vi "_goop4.llb_Interface_ViServerCall.vi"(8 "error in (no error)":errorcluster, 10 "Caller VI ref (This is the interface VI's reference)":refnum<vi>, 11 "Interface In":refnum<class>) -> (0 "error out":errorcluster, 3 "Interface Out":refnum<class>)   [LabVIEW 2014]
doc: "This VI handles the call to the overriding VI in the class that implements this interface.\nUse the \"This VI\" reference and wirre that to the Caller VI ref control."
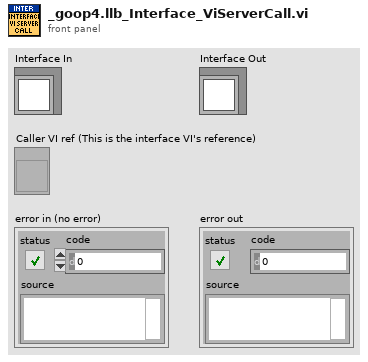
[diagram p1: front panel]
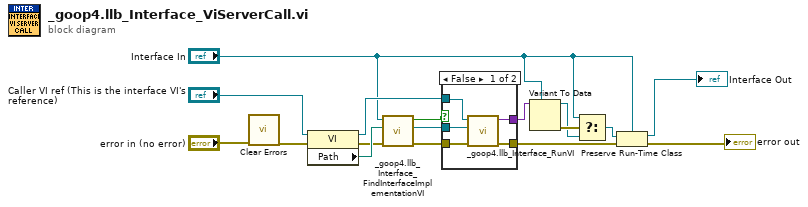
[diagram p0: block diagram]
diagram:
  n1 = call <vilib>:"Clear Errors.vi"("error in (no error)"="error in (no error)") -> ("error out"=w2:errorcluster)  [unwired: 5 in, 1 out]
  n2 = property class="VI"(reference="Caller VI ref (This is the interface VI's reference)", error in=w2) -> (reference out=w8:refnum<vi>, error out=w13:errorcluster, "Path"=w15:path)
  n3 = call "_goop4.llb_Interface_FindInterfaceImplementationVI.vi"("error in (no error)"=w13, "Path"=w15, "LabVIEW Object in"="Interface In") -> ("error out"=w14:errorcluster, "VI Refnum Of Interface method in class"=w7:refnum<vi>, "NoImplementationFound"=w6:bool)  [unwired: 5 in, 1 out]
  n4 = case shown="False" w6 {
    tunnel: [w20 w23] -> w4
    tunnel: w14 -> [w21 w23]
    tunnel: [w22 _] -> w17
    tunnel: w7 -> [w19 _]
    tunnel: w8 -> [w18 _]
    frame False {
      n5 = call "_goop4.llb_Interface_RunVI.vi"("error in (no error)"=w21, "VI of LvClass that implements this interface VI"=w19, "Interface VI"=w18) -> ("error out"=w20:errorcluster, "LvClassObjectDataOut(If the VI has a LVClass Indicator)"=w22:variant)  [unwired: 7 in]
    }
    frame True {
    }
  }
  n6 = Variant To Data(type="Interface In", Variant=w17) -> (data=w11:refnum<class>, error out=w12:errorcluster)  [unwired: 1 in]
  n7 = Select(t="Interface In", s=w12, f=w11) -> (s? t:f=w10:refnum<class>)
  n8 = Preserve Run-Time Class(object in=w10, error in=w4, 2:"Interface In") -> (object out=→"Interface Out":refnum<class>, error out=→"error out":errorcluster)
